vi "Convert to graph ranges.vi"(8 "Graph Ranges in":T2, 11 "Settings in":T1={"Name of test"="", "Date"=timestamp(0 s since 1904-01-01), "Location"="", "Template"="", "Soundcard"="", "resolution"=0, "Sampling rate"=0, "Ch1 Gain "=0.0, "Ch2 Gain"=0.0, "Sample time (s)"=0.0, "Pre-trigger (s)"=0.0, "Hammer Threshold"=0.0, "Positions"=0, "Taps/Position"=0, "Set Names"="", "Freq resolution"=0.0, "Hammer cutoff"=0.0, "Mic cutoff"=0.0, "Double bounce "=0.0, "Hammer Cal"=0.0, "dB Offset"=0.0, "Accel Cal"=0.0, "Vibrometer Cal"=0.0, "Mic Cal"=0.0, "Output"=0, "Voltage Cal"=0.0, "Vibrometer Port"="", "Range"=0, "High Pass"=0, "Bandwidth"=0, "X Range"=[], "Y Range"=[], "dB Spread"=0.0, "Trigger"=0, "Ch_1"=0, "Ch_2"=0, "flip?"=FALSE, "60Hz"=FALSE, "Time offset"=0.0, "Piezo Cal"=1.0, "Default Notes"=""} {"Ch_2" min=1 step=1; "Ch_1" min=1 max=100 step=1; "Trigger" items=["Hammer (force)", "Self-tap", "Spacebar"]; "Bandwidth" items=["1 kHz"=1, "5 kHz"=5, "10 kHz"=10, "25 kHz"=25, "50 kHz"=50, "100 kHz"=100]; "High Pass" items=["Off", "13 Hz", "104 Hz"]; "Range" items=["10 mm/s"=1, "20 mm/s"=2, "50 mm/s"=5, "100 mm/s"=10, "200 mm/s"=20, "500 mm/s"=50, "1 m/s"=100, "2 m/s"=200]; "Output" items=["Accelerometer", "Speed (from acceleration)", "Microphone", "Vibrometer", "Piezo"]; "Voltage Cal" format="%#_13g"; "Ch2 Gain" format="%#_13g"; "Ch1 Gain" format="%#_13g"; "Double bounce" min=0.0; "Mic cutoff" min=0.0 format="%#_4g"; "Hammer cutoff" min=0.0 format="%#_4g"; "Freq resolution" min=0.0; "Pre-trigger (s)" format="%#_13g"; "Date" format="%<%H:%M\n%d/%m/%y>T"; "resolution" items=["16 bit"=16, "24 bit"=24, "32 bit"=32]; "Sampling rate" items=["22050 samp/s"=22050, "44100 samp/s"=44100, "48000 samp/s"=48000]}) -> (0 "Settings out":T1={"Name of test"="", "Date"=timestamp(0 s since 1904-01-01), "Location"="", "Template"="", "Soundcard"="", "resolution"=32, "Sampling rate"=48000, "Ch1 Gain "=25.0, "Ch2 Gain"=10.0, "Sample time (s)"=0.3, "Pre-trigger (s)"=0.01, "Hammer Threshold"=10.0, "Positions"=12, "Taps/Position"=5, "Set Names"="", "Freq resolution"=10.0, "Hammer cutoff"=0.0, "Mic cutoff"=0.0, "Double bounce "=0.0, "Hammer Cal"=1.0, "dB Offset"=0.0, "Accel Cal"=1.0, "Vibrometer Cal"=1.0, "Mic Cal"=1.0, "Output"=2, "Voltage Cal"=1.0, "Vibrometer Port"="ASRL27::INSTR", "Range"=4, "High Pass"=2, "Bandwidth"=4, "X Range"=[], "Y Range"=[], "dB Spread"=0.0, "Trigger"=0, "Ch_1"=1, "Ch_2"=2, "flip?"=FALSE, "60Hz"=FALSE, "Time offset"=0.0, "Piezo Cal"=1.0, "Default Notes"=""} {"Ch_2" min=1 step=1; "Ch_1" min=1 max=100 step=1; "Trigger" items=["Hammer (force)", "Self-tap", "Spacebar"]; "Bandwidth" items=["1 kHz"=1, "5 kHz"=5, "10 kHz"=10, "25 kHz"=25, "50 kHz"=50, "100 kHz"=100]; "High Pass" items=["Off", "13 Hz", "104 Hz"]; "Range" items=["10 mm/s"=1, "20 mm/s"=2, "50 mm/s"=5, "100 mm/s"=10, "200 mm/s"=20, "500 mm/s"=50, "1 m/s"=100, "2 m/s"=200]; "Output" items=["Accelerometer", "Speed (from acceleration)", "Microphone", "Vibrometer", "Piezo"]; "Voltage Cal" format="%#_13g"; "Ch2 Gain" format="%#_13g"; "Ch1 Gain" format="%#_13g"; "Double bounce" min=0.0; "Mic cutoff" min=0.0 format="%#_4g"; "Hammer cutoff" min=0.0 format="%#_4g"; "Freq resolution" min=0.0; "Pre-trigger (s)" format="%#_13g"; "Date" format="%<%H:%M\n%d/%m/%y>T"; "resolution" items=["16 bit"=16, "24 bit"=24, "32 bit"=32]; "Sampling rate" items=["22050 samp/s"=22050, "44100 samp/s"=44100, "48000 samp/s"=48000]}, 3 "Graph Ranges out":T2)   [LabVIEW 2022 SP3]
uses:
  PreferencesControl.ctl
panel:
  # "Hz"
  # "dB"
  # "dB"
  # "sec"
  # "sec"
  # "mV/Pa"
  # "mV/m/s2"
  # "mV/mm/s"
  # "V/N"
  # "sec"
  # "sec"
  # "mV/N"
  # "a.u."
  # "a.u."
  # "sec"
  # "X Min      X Max      X Inc        X Minor   Y Min      Y Max       Y Inc        Y Minor"
  # "Hammer Spectrum\n\nHammer Level Meter \n\nMic Level Meter\n\nFreq Response Plot"
  # "Hz"
  # "dB"
  # "dB"
  # "sec"
  # "sec"
  # "mV/Pa"
  # "mV/m/s2"
  # "mV/mm/s"
  # "V/N"
  # "sec"
  # "sec"
  # "mV/N"
  # "a.u."
  # "a.u."
  # "sec"
  # "X Min      X Max      X Inc        X Minor   Y Min      Y Max       Y Inc        Y Minor"
  # "Hammer Spectrum\n\nHammer Level Meter \n\nMic Level Meter\n\nFreq Response Plot"
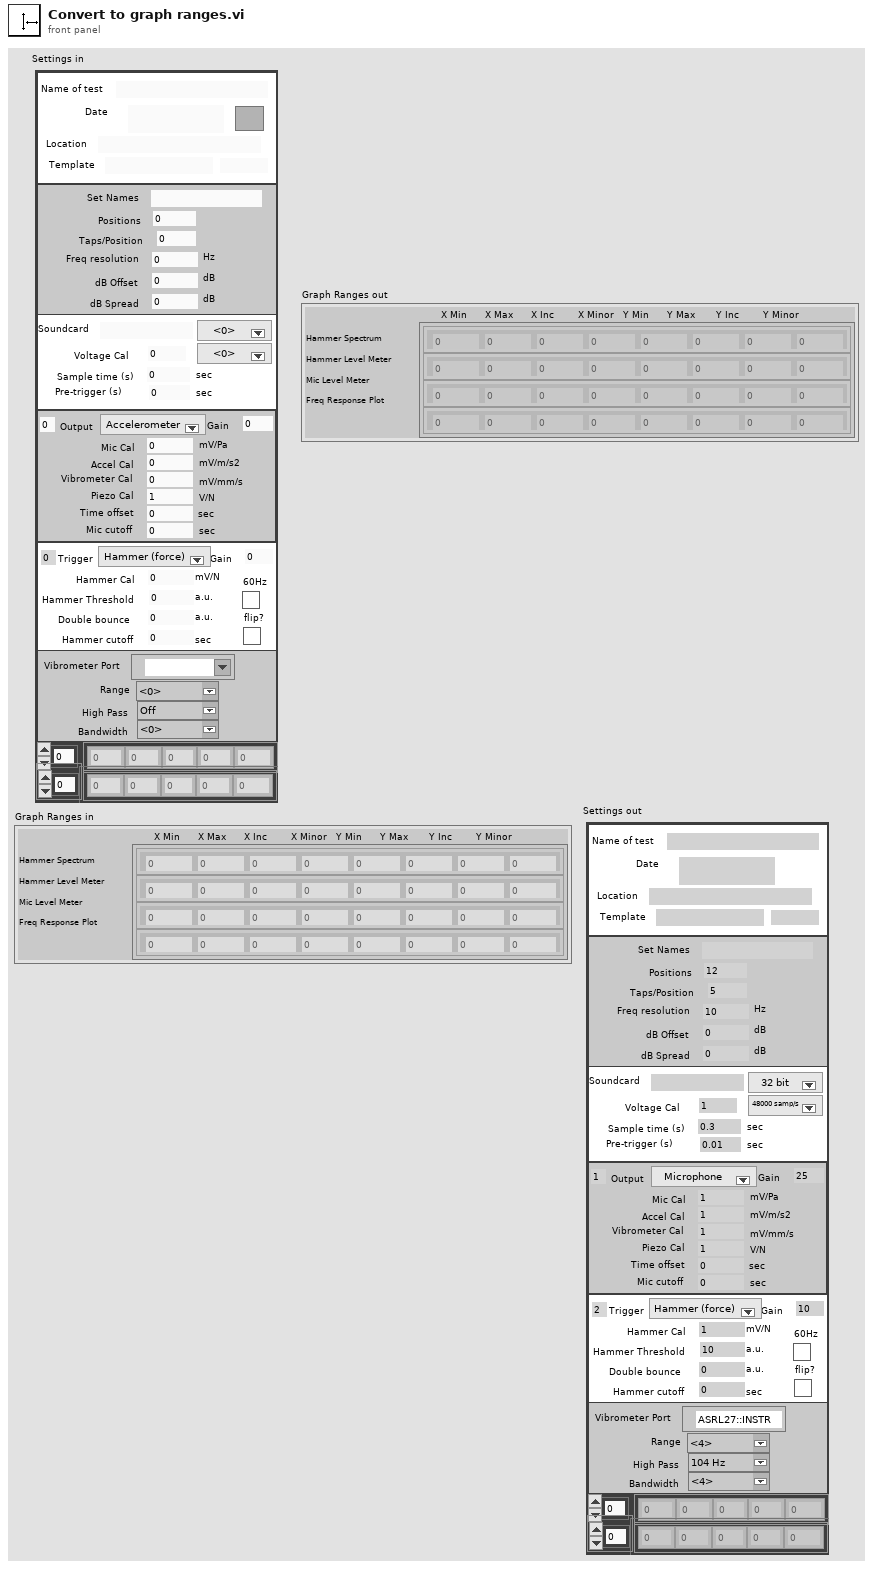
[diagram p1: front panel]
types:
  T1 = typedef "PreferencesControl.ctl" = cluster{"Name of test":string, "Date":timestamp, "Location":string, "Template":string, "Soundcard":string, "resolution":u16, "Sampling rate":u16, "Ch1 Gain ":dbl, "Ch2 Gain":dbl, "Sample time (s)":dbl, "Pre-trigger (s)":dbl, "Hammer Threshold":dbl, "Positions":i16, "Taps/Position":i16, "Set Names":string, "Freq resolution":dbl, "Hammer cutoff":dbl, "Mic cutoff":dbl, "Double bounce ":dbl, "Hammer Cal":dbl, "dB Offset":dbl, "Accel Cal":dbl, "Vibrometer Cal":dbl, "Mic Cal":dbl, "Output":u16, "Voltage Cal":dbl, "Vibrometer Port":refnum<visa-resource-name>, "Range":u16, "High Pass":u16, "Bandwidth":u16, "X Range":cluster{"Minimum":dbl, "Maximum":dbl, "Increment":dbl, "Minor Increment":dbl, "Start":dbl}[], "Y Range":cluster{"Minimum":dbl, "Maximum":dbl, "Increment":dbl, "Minor Increment":dbl, "Start":dbl}[], "dB Spread":dbl, "Trigger":u16, "Ch_1":u8, "Ch_2":u8, "flip?":bool, "60Hz":bool, "Time offset":dbl, "Piezo Cal":dbl, "Default Notes":string}
  T2 = cluster{"Ranges":cluster{"XMin":dbl, "XMax":dbl, "XInc":dbl, "XMinor":dbl, "YMin":dbl, "YMax":dbl, "YInc":dbl, "YMinor":dbl}[]}
  T3 = cluster{"Minimum":dbl, "Maximum":dbl, "Increment":dbl, "Minor Increment":dbl, "Start":dbl}[]
  T4 = cluster{"XMin":dbl, "XMax":dbl, "XInc":dbl, "XMinor":dbl, "YMin":dbl, "YMax":dbl, "YInc":dbl, "YMinor":dbl}[]
  T5 = cluster{"Minimum":dbl, "Maximum":dbl, "Increment":dbl, "Minor Increment":dbl, "Start":dbl}
  T6 = cluster{"Minimum":dbl, "Maximum":dbl, "Increment":dbl, "Minor Increment":dbl, "Minimum":dbl, "Maximum":dbl, "Increment":dbl, "Minor Increment":dbl}
  T7 = cluster{cluster{"Minimum":dbl, "Maximum":dbl, "Increment":dbl, "Minor Increment":dbl, "Minimum":dbl, "Maximum":dbl, "Increment":dbl, "Minor Increment":dbl}[]}
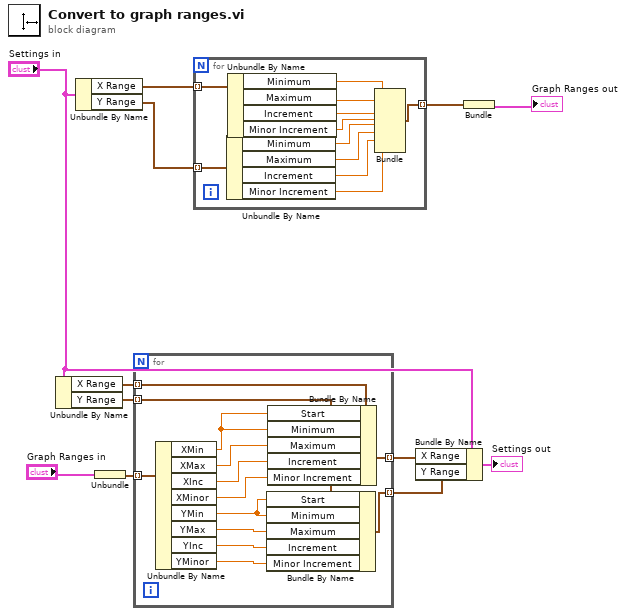
[diagram p0: block diagram]
diagram:
  n1 = Unbundle By Name("Settings in") -> ("X Range"=w8:T3, "Y Range"=w7:T3)
  n2 = Unbundle By Name("Settings in") -> ("X Range"=w9:T3, "Y Range"=w10:T3)
  n3 = Unbundle("Graph Ranges in") -> ("Ranges"=w3:T4)
  n4 = for {
    tunnel: w3 -> [w25] mode=indexing
    tunnel: w8 -> [w24] mode=indexing
    tunnel: w7 -> [w20] mode=indexing
    tunnel: [w22] -> w6 mode=indexing
    tunnel: [w21] -> w5 mode=indexing
    n5 = Unbundle By Name(w25) -> ("XMin"=w13:dbl, "XMax"=w23:dbl, "XInc"=w19:dbl, "XMinor"=w18:dbl, "YMin"=w14:dbl, "YMax"=w17:dbl, "YInc"=w16:dbl, "YMinor"=w15:dbl)
    n6 = Bundle By Name(cluster=w20, "Start"=w14, "Minimum"=w14, "Maximum"=w17, "Increment"=w16, "Minor Increment"=w15) -> (w21:T5)
    n7 = Bundle By Name(cluster=w24, "Start"=w13, "Minimum"=w13, "Maximum"=w23, "Increment"=w19, "Minor Increment"=w18) -> (w22:T5)
  }
  n8 = for {
    tunnel: w9 -> [w36] mode=indexing
    tunnel: w10 -> [w35] mode=indexing
    tunnel: [w31] -> w12 mode=indexing
    n9 = Unbundle By Name(w35) -> ("Minimum"=w28:dbl, "Maximum"=w33:dbl, "Increment"=w27:dbl, "Minor Increment"=w26:dbl)
    n10 = Unbundle By Name(w36) -> ("Minimum"=w34:dbl, "Maximum"=w32:dbl, "Increment"=w30:dbl, "Minor Increment"=w29:dbl)
    n11 = Bundle("Minimum"=w34, "Maximum"=w32, "Increment"=w30, "Minor Increment"=w29, "Minimum"=w28, "Maximum"=w33, "Increment"=w27, "Minor Increment"=w26) -> (w31:T6)  [unwired: 1 in]
  }
  n12 = Bundle By Name(cluster="Settings in", "X Range"=w6, "Y Range"=w5) -> (→"Settings out":T1)
  n13 = Bundle(w12) -> (→"Graph Ranges out":T7)  [unwired: 1 in]
